vi "clamp_protocol.vi"(3 "which clamp":enum16{"VClamp", "IClamp"}(ring), 4 "# reps":i32=10, 5 "# Iterations":i32, 6 "clamp in":T1, 7 "sampling rate (Hz)":i32) -> (0 "View profile (wvfrms)":waveform(dbl)[](graph), 1 "Stim profile":dbl[][](graph), 2 "samples to read":i32)   [LabVIEW 2019]
uses:
  Controls/clamp_profile.ctl
panel:
  out "size of resulting profile":i32[](array[numeric])
  out "View profile":dbl[][](graph)
  out "clamp out":T1
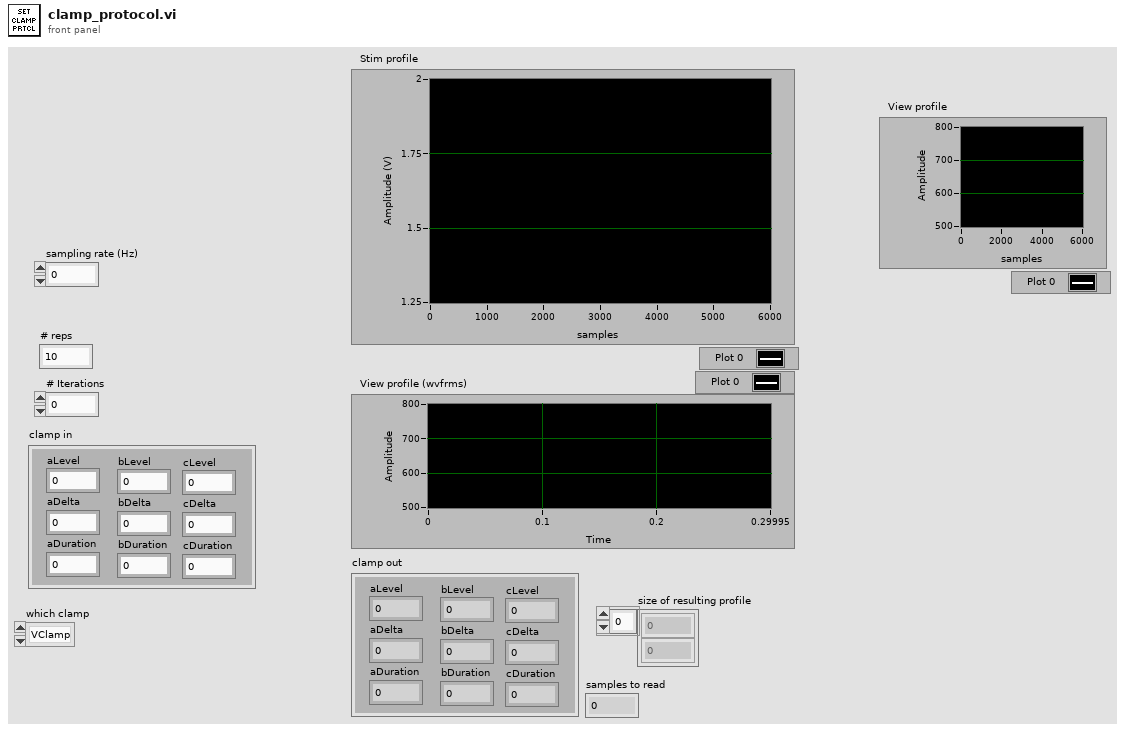
[diagram p1: front panel]
types:
  T1 = typedef "clamp_profile.ctl" = cluster{"aLevel":dbl, "aDelta":dbl, "aDuration":i32, "bLevel":dbl, "bDelta":dbl, "bDuration":i32, "cLevel":dbl, "cDelta":dbl, "cDuration":i32}
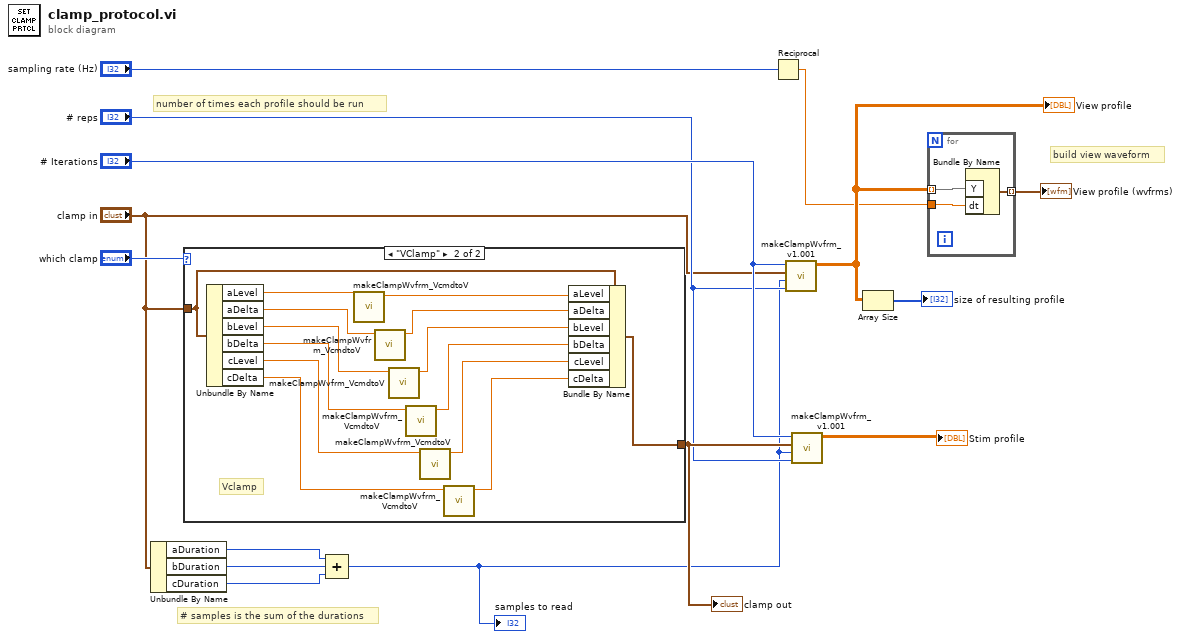
[diagram p0: block diagram]
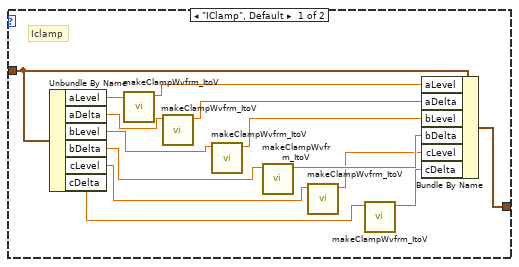
[diagram p2: hidden frame]
diagram:
  # "build view waveform"
  # "# samples is the sum of the durations"
  # "number of times each profile should be run"
  n1 = Unbundle By Name("clamp in") -> ("aDuration"=w8:i32, "bDuration"=w7:i32, "cDuration"=w6:i32)
  n2 = case shown="\"VClamp\"" "which clamp" {
    tunnel: "clamp in" -> [w23 w43]
    tunnel: [w16 w42] -> w14
    frame "IClamp", Default {
      # "Iclamp"
      n3 = Unbundle By Name(w23) -> ("aLevel"=w29:dbl, "aDelta"=w28:dbl, "bLevel"=w27:dbl, "bDelta"=w26:dbl, "cLevel"=w25:dbl, "cDelta"=w24:dbl)
      n4 = call "makeClampWvfrm_ItoV.vi"("Current in (pA)"=w29) -> ("cmd voltage (V)"=w22:dbl)  [unwired: 10 in]
      n5 = call "makeClampWvfrm_ItoV.vi"("Current in (pA)"=w28) -> ("cmd voltage (V)"=w21:dbl)  [unwired: 10 in]
      n6 = call "makeClampWvfrm_ItoV.vi"("Current in (pA)"=w27) -> ("cmd voltage (V)"=w20:dbl)  [unwired: 10 in]
      n7 = call "makeClampWvfrm_ItoV.vi"("Current in (pA)"=w26) -> ("cmd voltage (V)"=w19:dbl)  [unwired: 10 in]
      n8 = call "makeClampWvfrm_ItoV.vi"("Current in (pA)"=w25) -> ("cmd voltage (V)"=w18:dbl)  [unwired: 10 in]
      n9 = call "makeClampWvfrm_ItoV.vi"("Current in (pA)"=w24) -> ("cmd voltage (V)"=w17:dbl)  [unwired: 10 in]
      n10 = Bundle By Name(cluster=w23, "aLevel"=w22, "aDelta"=w21, "bLevel"=w20, "bDelta"=w19, "cLevel"=w18, "cDelta"=w17) -> (w16:T1)
    }
    frame "VClamp" {
      # "Vclamp"
      n11 = Unbundle By Name(w43) -> ("aLevel"=w41:dbl, "aDelta"=w39:dbl, "bLevel"=w38:dbl, "bDelta"=w37:dbl, "cLevel"=w36:dbl, "cDelta"=w35:dbl)
      n12 = call "makeClampWvfrm_VcmdtoV.vi"("voltage in (mV)"=w41) -> ("cmd voltage (V)"=w40:dbl)  [unwired: 10 in]
      n13 = call "makeClampWvfrm_VcmdtoV.vi"("voltage in (mV)"=w39) -> ("cmd voltage (V)"=w34:dbl)  [unwired: 10 in]
      n14 = call "makeClampWvfrm_VcmdtoV.vi"("voltage in (mV)"=w38) -> ("cmd voltage (V)"=w33:dbl)  [unwired: 10 in]
      n15 = call "makeClampWvfrm_VcmdtoV.vi"("voltage in (mV)"=w37) -> ("cmd voltage (V)"=w32:dbl)  [unwired: 10 in]
      n16 = call "makeClampWvfrm_VcmdtoV.vi"("voltage in (mV)"=w36) -> ("cmd voltage (V)"=w31:dbl)  [unwired: 10 in]
      n17 = call "makeClampWvfrm_VcmdtoV.vi"("voltage in (mV)"=w35) -> ("cmd voltage (V)"=w30:dbl)  [unwired: 10 in]
      n18 = Bundle By Name(cluster=w43, "aLevel"=w40, "aDelta"=w34, "bLevel"=w33, "bDelta"=w32, "cLevel"=w31, "cDelta"=w30) -> (w42:T1)
    }
  }
  "clamp out" <- w14
  n19 = Compound Arithmetic op=ADD(w8, w7, w6) -> (w5:i32)
  "samples to read" <- w5
  n20 = Reciprocal(x="sampling rate (Hz)") -> (1/x=w2:dbl)
  n21 = call "makeClampWvfrm_v1.001.vi"("# reps"="# reps", "Samples to Read"=w5, "clamp in"="clamp in", "# Iterations"="# Iterations") -> ("Array"=w4:dbl[][])  [unwired: 7 in]
  "View profile" <- w4
  n22 = call "makeClampWvfrm_v1.001.vi"("# reps"="# reps", "Samples to Read"=w5, "clamp in"=w14, "# Iterations"="# Iterations") -> ("Array"=→"Stim profile":dbl[][])  [unwired: 7 in]
  n23 = Array Size(array=w4) -> (size(s)=→"size of resulting profile":i32[])
  n24 = for {
    tunnel: w4 -> [w46] mode=indexing
    tunnel: [w45] -> w1 mode=indexing
    tunnel: w2 -> [w44]
    n25 = Bundle By Name("Y"=w46, "dt"=w44) -> (w45:waveform(dbl))  [unwired: 1 in]
  }
  "View profile (wvfrms)" <- w1
